vi "Test 082021.vi"() -> ()   [LabVIEW 2019]
uses:
  <vilib>/Utility/error.llb/DialogType.ctl
  <vilib>/DAQmx/write.llb/DAQmx Write (Analog 1D Wfm NChan NSamp).vi
  <vilib>/DAQmx/read.llb/DAQmx Read (Analog 2D DBL NChan NSamp).vi
  <vilib>/DAQmx/create/channels.llb/DAQmx Create Channel (AO-Voltage-Basic).vi
  <vilib>/DAQmx/configure/timing.llb/DAQmx Timing (Sample Clock).vi
  <vilib>/DAQmx/configure/trigger.llb/DAQmx Start Trigger (Digital Edge).vi
  <vilib>/DAQmx/configure/trigger.llb/DAQmx Start Trigger (Time).vi
  <vilib>/DAQmx/configure/trigger.llb/DAQmx Start Trigger (Analog Edge).vi
  <vilib>/DAQmx/miscellaneous.llb/DAQmx Fill In Error Info.vi
  <vilib>/DAQmx/create/channels.llb/DAQmx Create Channel (AI-Voltage-Basic).vi
  <vilib>/DAQmx/configure/trigger.llb/DAQmx Reference Trigger (Digital Edge).vi
  <resource>/objmgr/daqmx.rc
  <vilib>/measure/NI_MABase.lvlib
panel:
  in  "AI pretrigger samples per channel":u32=2
  in  "AI Trigger Edge":i32(ring)=10280 items=["Rising"=10280, "Falling"=10171]
  in  "AI Trigger Source":tag="/cDAQ1/ao/SampleClock"
  out "AI SampClk.Rate":dbl=1000000.0
  in  "AI Clock Source":tag="OnboardClock"
  out "Waveform Graph 2":dbl[][](graph)
  in  "physical channels":tag="cDAQ1Mod1/ai0:3"
  in  "Trigger Type":T1(tab)
  in  "Digital Start Trigger Edge":i32(ring)=10280 caption="Edge" items=["Rising"=10280, "Falling"=10171]
  in  "Digital Start Trigger Source":tag="/Dev1/PFI0" caption="Source"
  in  "Digital Pause Trigger Pause When":i32(ring)=10192 caption="Pause When" items=["High"=10192, "Low"=10214]
  in  "Digital Pause Trigger Source":tag="/Dev1/PFI0" caption="Source"
  in  "Analog Start Trigger Level":dbl caption="Level" format="%0.2f"
  in  "Analog Start Trigger Hysteresis":dbl caption="Hysteresis" format="%.2f"
  in  "Analog Start Trigger Slope":i32(ring)=10280 caption="Slope" items=["Rising"=10280, "Falling"=10171]
  in  "Analog Start Trigger Source":string="APFI0" caption="Source"
  in  "Analog Pause Trigger Source":string="APFI0" caption="Source"
  in  "Analog Pause Trigger Pause When":i32(ring)=10093 caption="Pause When" items=["Above Level"=10093, "Below Level"=10107]
  in  "Analog Pause Trigger Level":dbl caption="Level" format="%.2f"
  in  "When":timestamp
  in  "Select Time\nManually":bool
  out "Waveform Graph":waveform(dbl)[](graph)
  in  "Output Array":T2(array[cluster])=[{"Waveform Type"=0, "Amplitude"=1.0, "Frequency"=1200.0}] {"Frequency" format="%0.2p"; "Amplitude" format="%0.2p"; "Waveform Type" items=["Sine Wave", "Triangle Wave", "Square Wave", "Sawtooth Wave"]}
  in  "Number of Samples":i32=7000000
  in  "Sample Rate":dbl=1000000.0
  in  "AO Sample Clock Source":tag="OnboardClock"
  in  "Max Voltage":dbl=5.0
  in  "Min Voltage":dbl=-5.0
  in  "Physical Channel(s)":tag="cDAQ1Mod2/ao0"
  out "Actual Sample Rate":dbl=1000000.0 format="%0.2f"
  # "To enable triggers, select a tab above, and configure the settings.\n\nNot all hardware supports all trigger types. Refer to your device documentation for more information."
  # "This trigger type is not supported in output tasks. \n\nRefer to your device documentation for more information on which triggers are supported."
  # "This trigger type is not supported in output tasks. \n\nRefer to your device documentation for more information on which triggers are supported."
  # "If time is not manually set, task will begin after 10 seconds"
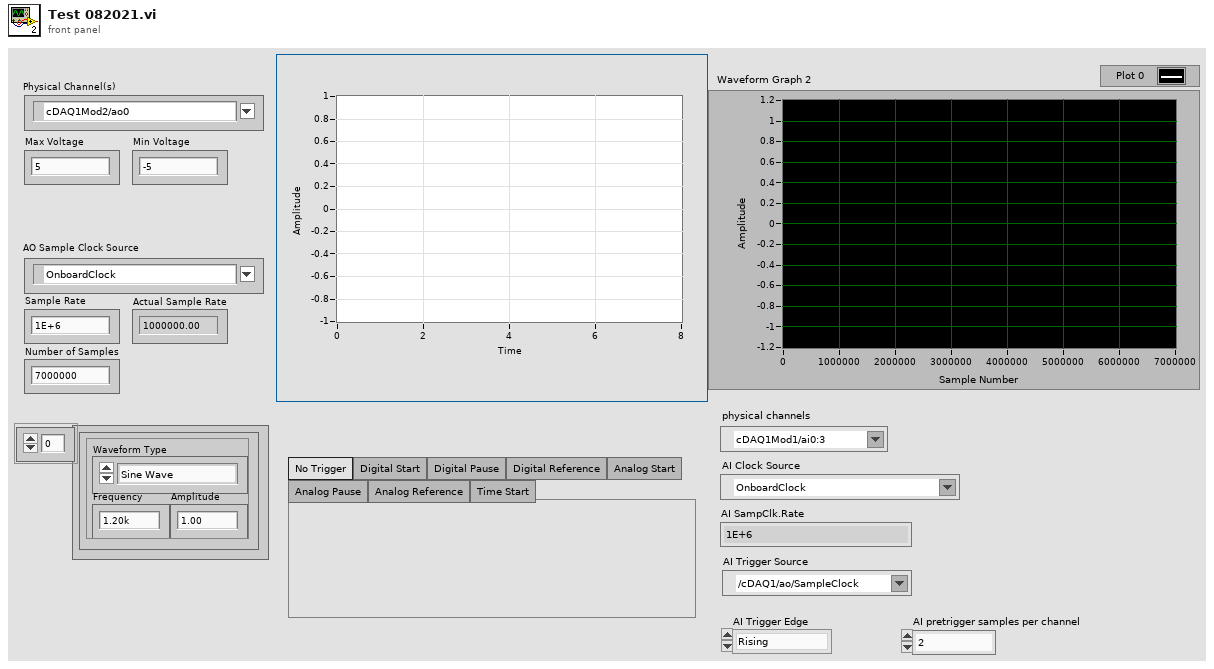
[diagram p1: front panel]
types:
  T1 = enum32{"No Trigger", "Digital Start", "Digital Pause", "Digital Reference", "Analog Start", "Analog Pause", "Analog Reference", "Time Start"}
  T2 = cluster{"Waveform Type":u16, "Amplitude":dbl, "Frequency":dbl}[]
  T3 = typedef "DialogType.ctl" = u16
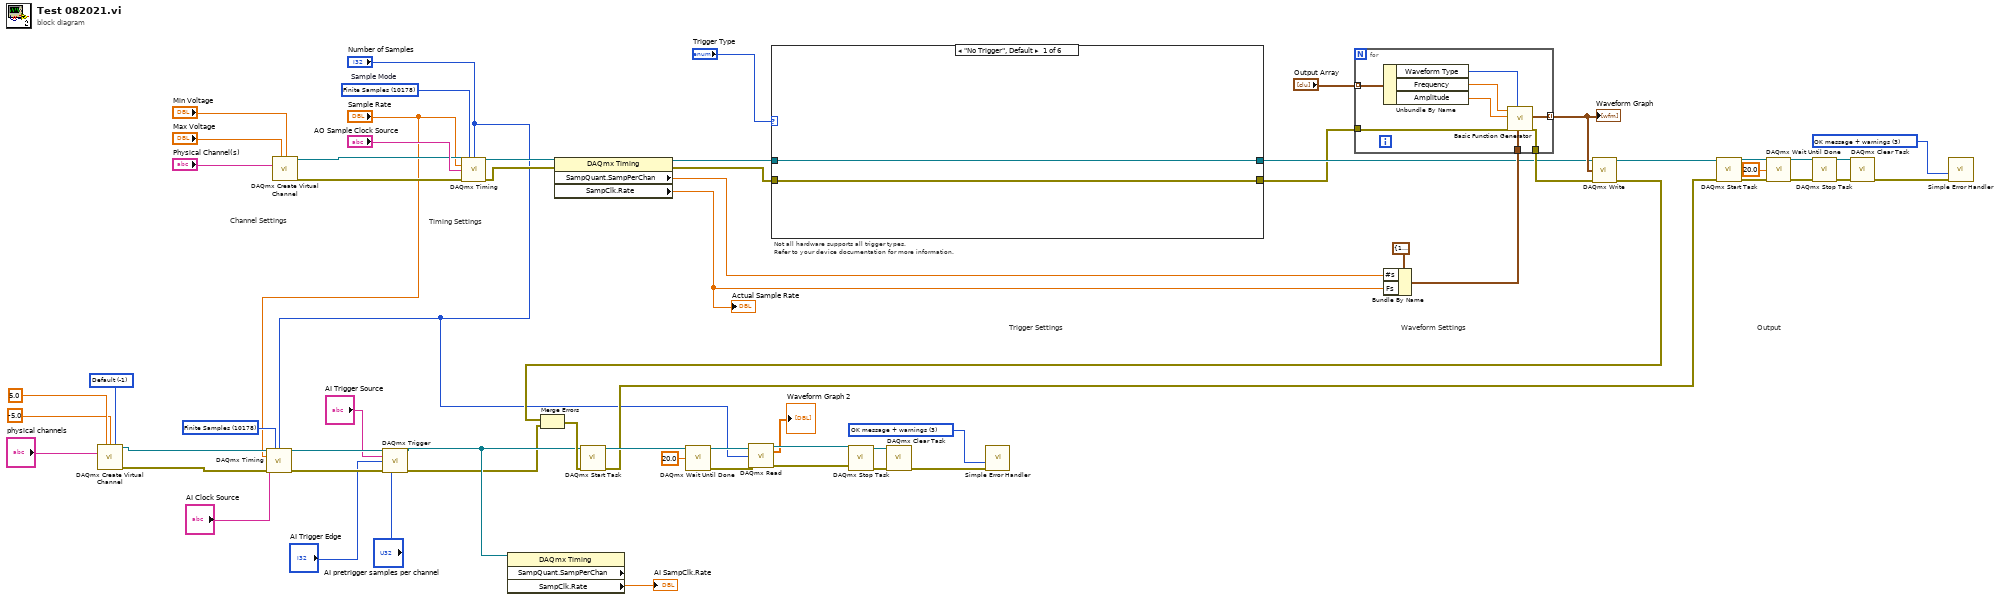
[diagram p0: block diagram]
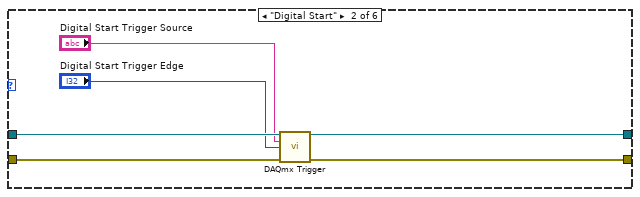
[diagram p2: hidden frame]
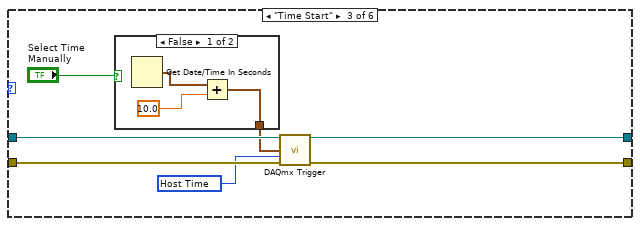
[diagram p3: hidden frame]
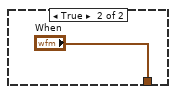
[diagram p4: hidden frame]
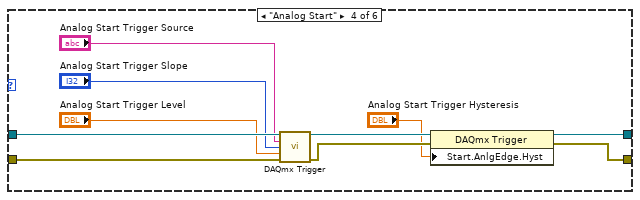
[diagram p5: hidden frame]
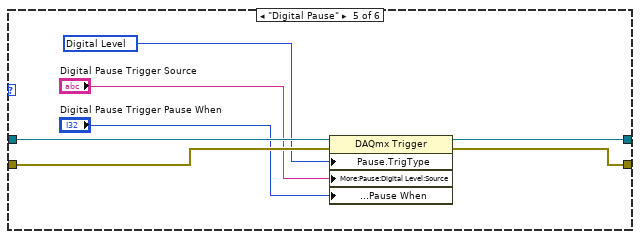
[diagram p6: hidden frame]
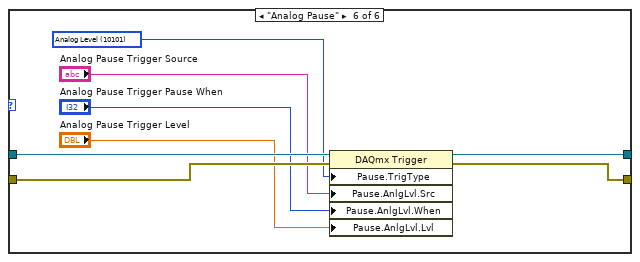
[diagram p7: hidden frame]
diagram:
  w18 = 10178 items=["Finite Samples"=10178, "Continuous Samples"=10123, "Hardware Timed Single Point"=12522] ("sample mode")
  w26 = T3 3 items=["no dialog", "OK message", "continue or stop message", "OK message + warnings", "continue/stop + warnings"] ("type of dialog (OK msg:1)")
  w31 = -1 items=["Default"=-1, "RSE"=10083, "NRSE"=10078, "Differential"=10106, "Pseudodifferential"=12529] ("input terminal configuration")
  w41 = T3 3 items=["no dialog", "OK message", "continue or stop message", "OK message + warnings", "continue/stop + warnings"] ("type of dialog (OK msg:1)")
  w61 = 10178 items=["Finite Samples"=10178, "Continuous Samples"=10123, "Hardware Timed Single Point"=12522]  # Sample Mode
  # "Trigger Settings"
  # "Not all hardware supports all trigger types.\nRefer to your device documentation for more information."
  # "Output"
  # "Waveform Settings"
  # "Timing Settings"
  # "Channel Settings"
  n1 = call-poly <vilib>:"DAQmx Create Virtual Channel.vi"("maximum value"=5.0, "minimum value"=-5.0, "input terminal configuration"=w31, "physical channels"="physical channels") -> ("task out"=w25:refnum<k21>, "error out"=w22:errorcluster)  [unwired: 10 in]
  n2 = call-poly <vilib>:"DAQmx Timing.vi"("task/channels in"=w25, "sample mode"=w18, "samples per channel"="Number of Samples", "rate"="Sample Rate", "source"="AI Clock Source", "error in"=w22) -> ("task out"=w10:refnum<k21>, "error out"=w8:errorcluster)  [unwired: 8 in]
  n3 = call-poly <vilib>:"DAQmx Create Virtual Channel.vi"("maximum value"="Max Voltage", "minimum value"="Min Voltage", "physical channels"="Physical Channel(s)") -> ("task out"=w35:refnum<k21>, "error out"=w60:errorcluster)  [unwired: 11 in]
  n4 = call-poly <vilib>:"DAQmx Trigger.vi"("task/channels in"=w10, "source"="AI Trigger Source", "edge"="AI Trigger Edge", "error in"=w8, "pretrigger samples per channel"="AI pretrigger samples per channel") -> ("task out"=w9:refnum<k21>, "error out"=w7:errorcluster)  [unwired: 9 in]
  n5 = call-poly <vilib>:"DAQmx Timing.vi"("task/channels in"=w35, "sample mode"=w61, "samples per channel"="Number of Samples", "rate"="Sample Rate", "source"="AO Sample Clock Source", "error in"=w60) -> ("task out"=w63:refnum<k21>, "error out"=w62:errorcluster)  [unwired: 8 in]
  n6 = property class="DAQmx Timing" props=["SampQuant.SampPerChan", "SampClk.Rate"](reference=w9) -> ("SampClk.Rate"=→"AI SampClk.Rate":dbl)  [unwired: 1 in, 3 out]
  n7 = property class="DAQmx Timing"(reference=w63, error in=w62) -> (reference out=w36:refnum<k21>, error out=w37:errorcluster, "SampQuant.SampPerChan"=w46:dbl, "SampClk.Rate"=w19:dbl)
  "Actual Sample Rate" <- w19
  n8 = case shown="\"No Trigger\", Default" "Trigger Type" {
    tunnel: w36 -> [w65 w71 w78 w92 w99 w107]
    tunnel: w37 -> [w64 w70 w77 w91 w96 w104]
    tunnel: [w65 w69 w76 w89 w98 w106] -> w39
    tunnel: [w64 w68 w75 w88 w97 w105] -> w38
    frame "No Trigger", Default {
    }
    frame "Digital Start" {
      n9 = call-poly <vilib>:"DAQmx Trigger.vi"("task/channels in"=w71, "source"="Digital Start Trigger Source", "edge"="Digital Start Trigger Edge", "error in"=w70) -> ("task out"=w69:refnum<k21>, "error out"=w68:errorcluster)  [unwired: 10 in]
    }
    frame "Time Start" {
      w74 = 16126 items=["Host Time"=16126, "I/O Device Time"=16127] ("timescale")
      n10 = case shown="False" "Select Time\nManually" {
        tunnel: [w80 "When"] -> w72
        frame False {
          n11 = Get Date/Time In Seconds() -> (seconds since 1Jan1904=w81:timestamp)
          n12 = Add(x=w81, y=10.0) -> (x+y=w80:timestamp)
        }
        frame True {
        }
      }
      n13 = call-poly <vilib>:"DAQmx Trigger.vi"("task/channels in"=w78, "when"=w72, "timescale"=w74, "error in"=w77) -> ("task out"=w76:refnum<k21>, "error out"=w75:errorcluster)  [unwired: 10 in]
    }
    frame "Analog Start" {
      n14 = call-poly <vilib>:"DAQmx Trigger.vi"("task/channels in"=w92, "source"="Analog Start Trigger Source", "slope"="Analog Start Trigger Slope", "level"="Analog Start Trigger Level", "error in"=w91) -> ("task out"=w87:refnum<k21>, "error out"=w86:errorcluster)  [unwired: 9 in]
      n15 = property class="DAQmx Trigger"(reference=w87, error in=w86, "Start.AnlgEdge.Hyst"="Analog Start Trigger Hysteresis") -> (reference out=w89:refnum<k21>, error out=w88:errorcluster)
    }
    frame "Digital Pause" {
      w95 = 10152 items=["Analog Level"=10101, "Analog Window"=10103, "Digital Level"=10152, "Digital Pattern"=10398, "None"=10230] ("Pause.TrigType")
      n16 = property class="DAQmx Trigger"(reference=w99, error in=w96, "Pause.TrigType"=w95, "More:Pause:Digital Level:Source"="Digital Pause Trigger Source", "More:Pause:Digital Level:Pause When"="Digital Pause Trigger Pause When") -> (reference out=w98:refnum<k21>, error out=w97:errorcluster)
    }
    frame "Analog Pause" {
      w103 = 10101 items=["Analog Level"=10101, "Analog Window"=10103, "Digital Level"=10152, "Digital Pattern"=10398, "None"=10230] ("Pause.TrigType")
      n17 = property class="DAQmx Trigger"(reference=w107, error in=w104, "Pause.TrigType"=w103, "Pause.AnlgLvl.Src"="Analog Pause Trigger Source", "Pause.AnlgLvl.When"="Analog Pause Trigger Pause When", "Pause.AnlgLvl.Lvl"="Analog Pause Trigger Level") -> (reference out=w106:refnum<k21>, error out=w105:errorcluster)
    }
  }
  n18 = Bundle By Name(cluster=cluster{"Fs":dbl, "#s":dbl} {"Fs"=1000.0, "#s"=1000.0} ("sampling info"), "#s"=w46, "Fs"=w19) -> (w53:cluster{"Fs":dbl, "#s":dbl})
  n19 = for {
    tunnel: w38 -> [w115]
    tunnel: w53 -> [w114]
    tunnel: [w113] -> w51
    tunnel: "Output Array" -> [w112] mode=indexing
    tunnel: [w108] -> w49 mode=indexing
    n20 = Unbundle By Name(w112) -> ("Waveform Type"=w111:u16, "Frequency"=w110:dbl, "Amplitude"=w109:dbl)
    n21 = call <vilib>:"Basic Function Generator.vi"("sampling info"=w114, "signal type"=w111, "error in (no error)"=w115, "amplitude"=w109, "frequency"=w110) -> ("error out"=w113:errorcluster, "signal out"=w108:waveform(dbl))  [unwired: 4 in, 1 out]
  }
  "Waveform Graph" <- w49
  n22 = call-poly <vilib>:"DAQmx Write.vi"("task/channels in"=w39, "data"=w49, "error in"=w51) -> ("task out"=w52:refnum<k21>, "error out"=w16:errorcluster)  [unwired: 10 in, 1 out]
  n23 = Merge Errors(w16, w7) -> (w15:errorcluster)
  n24 = call <vilib>:"DAQmx Start Task.vi"("task/channels in"=w9, "error in"=w15) -> ("task out"=w29:refnum<k21>, "error out"=w14:errorcluster)  [unwired: 12 in]
  n25 = call <vilib>:"DAQmx Wait Until Done.vi"("task/channels in"=w29, "timeout (sec)"=20.0) -> ("task out"=w24:refnum<k21>, "error out"=w21:errorcluster)  [unwired: 12 in]
  n26 = call-poly <vilib>:"DAQmx Read.vi"("task/channels in"=w24, "number of samples per channel"="Number of Samples", "error in"=w21) -> ("task out"=w23:refnum<k21>, "data"=→"Waveform Graph 2":dbl[][], "error out"=w20:errorcluster)  [unwired: 10 in]
  n27 = call <vilib>:"DAQmx Stop Task.vi"("task/channels in"=w23, "error in"=w20) -> ("task out"=w28:refnum<k21>, "error out"=w27:errorcluster)  [unwired: 12 in]
  n28 = call <vilib>:"DAQmx Clear Task.vi"("task in"=w28, "error in"=w27) -> ("error out"=w30:errorcluster)  [unwired: 13 in]
  n29 = call <vilib>:"Simple Error Handler.vi"("type of dialog (OK msg:1)"=w26, "error in (no error)"=w30) -> ()  [unwired: 3 in, 5 out]
  n30 = call <vilib>:"DAQmx Start Task.vi"("task/channels in"=w52, "error in"=w14) -> ("task out"=w48:refnum<k21>, "error out"=w47:errorcluster)  [unwired: 12 in]
  n31 = call <vilib>:"DAQmx Wait Until Done.vi"("task/channels in"=w48, "timeout (sec)"=20.0, "error in"=w47) -> ("task out"=w43:refnum<k21>, "error out"=w42:errorcluster)  [unwired: 11 in]
  n32 = call <vilib>:"DAQmx Stop Task.vi"("task/channels in"=w43, "error in"=w42) -> ("task out"=w45:refnum<k21>, "error out"=w44:errorcluster)  [unwired: 12 in]
  n33 = call <vilib>:"DAQmx Clear Task.vi"("task in"=w45, "error in"=w44) -> ("error out"=w59:errorcluster)  [unwired: 13 in]
  n34 = call <vilib>:"Simple Error Handler.vi"("type of dialog (OK msg:1)"=w41, "error in (no error)"=w59) -> ()  [unwired: 3 in, 5 out]
